vi "Write PID.vi"(8 "error in (no error)":errorcluster, 10 "PID":string, 11 "BuildWorker Controller in":refnum<class "BuildWorker Controller.lvclass">) -> (0 "error out":errorcluster, 3 "BuildWorker Controller out":refnum<class "BuildWorker Controller.lvclass">)   [LabVIEW 2017, in "BuildWorker Interface.lvlib" / "BuildWorker Controller.lvclass"]
uses:
  BuildWorker Controller.lvclass
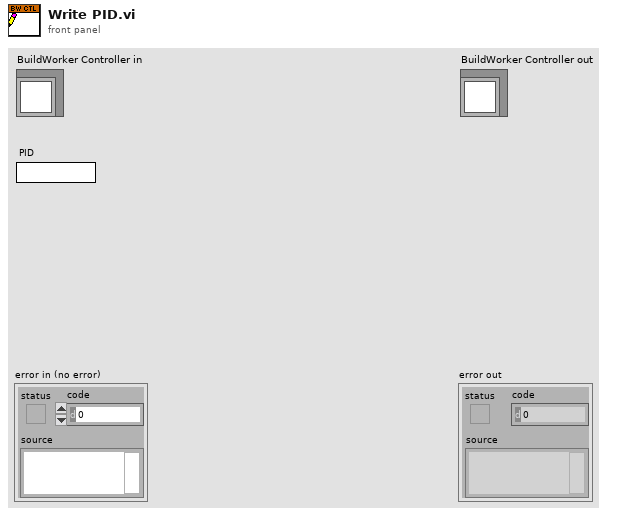
[diagram p1: front panel]
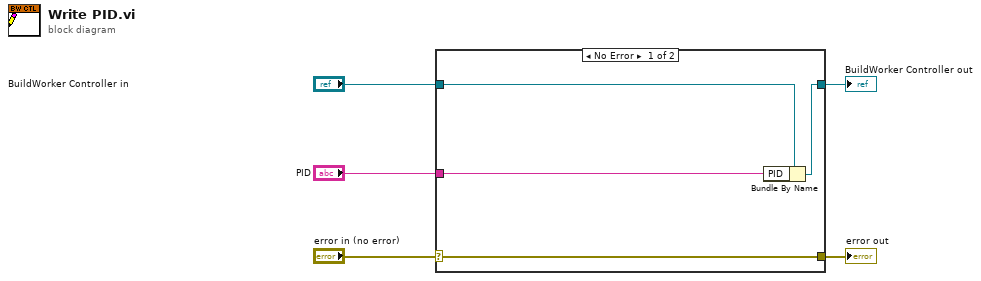
[diagram p0: block diagram]
diagram:
  n1 = case shown="No Error" "error in (no error)" {
    selector: "error in (no error)" -> [w9 w10]
    tunnel: [w9 w10] -> w4
    tunnel: [w7 w11] -> w2
    tunnel: "BuildWorker Controller in" -> [w8 w11]
    tunnel: "PID" -> [w6 _]
    frame No Error {
      n2 = Bundle By Name(cluster=w8, "PID"=w6) -> (w7:refnum<class "BuildWorker Controller.lvclass">)
    }
    frame Error {
    }
  }
  "error out" <- w4
  "BuildWorker Controller out" <- w2
